vi "Send Message.vi"(7 "Response Type (None)":refnum<class "Response.lvclass">, 8 "error in (no error)":errorcluster, 9 "timeout in ms (1000)":i32=1000, 10 "Client Message":refnum<class "Client Message.lvclass">, 11 "OBS in":refnum<class "OBS.lvclass">) -> (0 "error out":errorcluster, 1 "Has Response?":bool, 2 "Response":refnum<class "Response.lvclass">, 3 "OBS out":refnum<class "OBS.lvclass">)   [LabVIEW 2022 SP3, in "obs-websocket-lv.lvlib" / "OBS.lvclass"]
uses:
  OBS.lvclass
  Client Message/Client Message.lvclass
  Response/Response.lvclass
  Client Message.ctl
  OBS.lvclass/OBS.ctl
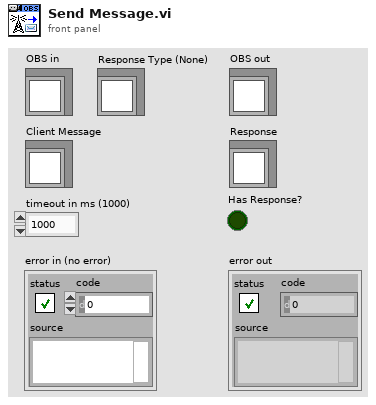
[diagram p1: front panel]
types:
  T1 = typedef "obs-websocket-lv.lvlib/OBS.lvclass/Client Message.ctl" = cluster{"Message":refnum<class "Client Message.lvclass">, "Response Notifier":refnum<notifier>}
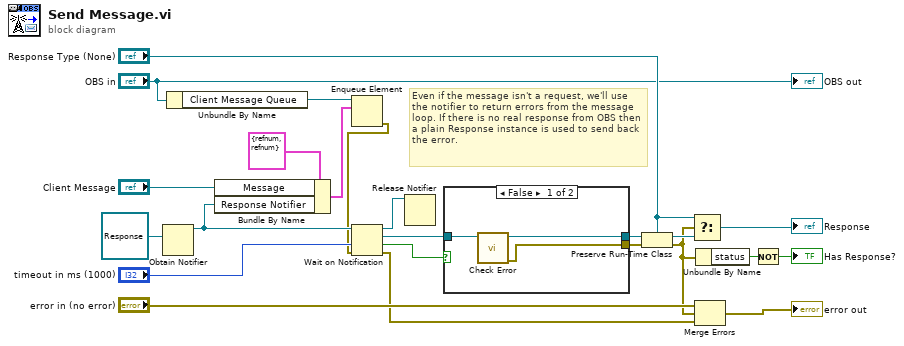
[diagram p0: block diagram]
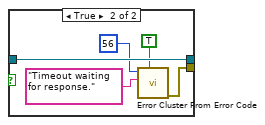
[diagram p2: hidden frame]
diagram:
  # "Even if the message isn't a request, we'll use the notifier to return errors from the message loop. If there is no real response from OBS then a plain Response instance is used to send back the error."
  n1 = Obtain Notifier(notification data type=refnum<class "Response.lvclass"> refnum ("obs-websocket-lv.lvlib:Response.lvclass")) -> (notifier out=w9:refnum<notifier>)  [unwired: 3 in, 2 out]
  n2 = Unbundle By Name("OBS in") -> ("Client Message Queue"=w11:refnum<queue>)
  n3 = Bundle By Name(cluster=T1 {"Message"=refnum, "Response Notifier"=refnum} ("Client Message"), "Message"="Client Message", "Response Notifier"=w9) -> (w10:T1)
  n4 = Enqueue Element(queue=w11, element=w10) -> (error out=w2:errorcluster)  [unwired: 2 in, 2 out]
  n5 = Wait on Notification(notifier=w9, timeout in ms (-1)="timeout in ms (1000)", error in (no error)=w2) -> (notifier out=w5:refnum<notifier>, notification=w6:refnum<class "Response.lvclass">, timed out?=w7:bool, error out=w1:errorcluster)  [unwired: 1 in]
  n6 = Release Notifier(notifier=w5) -> ()  [unwired: 2 in, 3 out]
  n7 = case shown="False" w7 {
    tunnel: w6 -> [w24 w30]
    tunnel: [w26 w31] -> w4
    tunnel: [w25 w30] -> w3
    frame False {
      n8 = call "Check Error.vi"("Response in"=w24) -> ("error out"=w26:errorcluster, "Response out"=w25:refnum<class "Response.lvclass">)  [unwired: 9 in]
    }
    frame True {
      n9 = call <vilib>:"Error Cluster From Error Code.vi"("show call chain? (False)"=TRUE, "error message (\"\")"="Timeout waiting for response." ("error message (\"\")"), "error code (0)"=56) -> ("error out"=w31:errorcluster)  [unwired: 6 in]
    }
  }
  n10 = Preserve Run-Time Class(object in=w3, error in=w4, 2:"Response Type (None)") -> (object out=w18:refnum<class "Response.lvclass">, error out=w16:errorcluster)
  n11 = Select(t="Response Type (None)", s=w16, f=w18) -> (s? t:f=→"Response":refnum<class "Response.lvclass">)
  n12 = Merge Errors("error in (no error)", w16, w1) -> (→"error out":errorcluster)
  n13 = Unbundle By Name(w16) -> ("status"=w21:bool)
  n14 = Not(x=w21) -> (.not. x?=→"Has Response?":bool)
  "OBS out" <- "OBS in"
